vi "create Behaviour.vi"(8 "error in (no error)":errorcluster caption="Fehler (Eingang, kein Fehler)", 11 "TestInterface Eingang":refnum<class "TestInterface.lvclass"> caption="DNL_LabVIEW Object in") -> (0 "error out":errorcluster caption="Fehler (Ausgang)", 1 "regex":string[](array[string]), 2 "response":bool[](array[boolean]), 3 "TestInterface Ausgang":refnum<class "TestInterface.lvclass"> caption="DNL_LabVIEW Object out")   [LabVIEW 2013, in "TestInterface.lvclass"]
doc: "In diesem VI werden die beiden Arrays regex und response für das Verhalten festgelegt. Das Array response definiert, ob eine Antwort auf einen Befehl erwartet wird oder nicht. Die Erstellung des Verhaltens ist hardcoded und wird nicht während der Laufzeit erstellt."
uses:
  TestInterface.lvclass
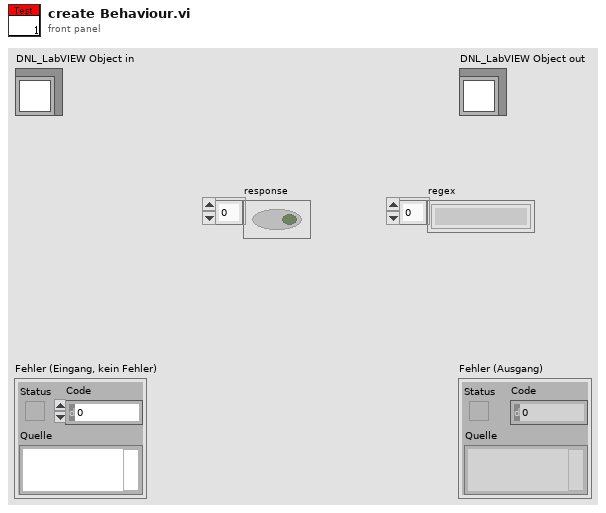
[diagram p1: front panel]
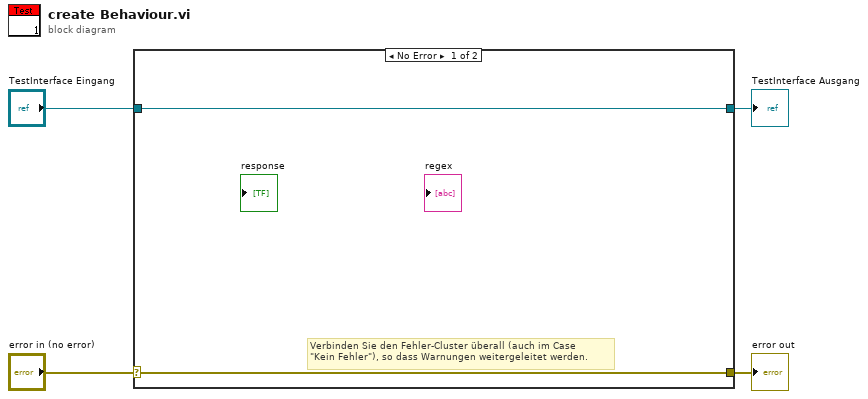
[diagram p0: block diagram]
diagram:
  n1 = case shown="No Error" "error in (no error)" {
    selector: "error in (no error)" -> [w5 w8]
    tunnel: [w5 w8] -> w3
    tunnel: [w6 w7] -> w1
    tunnel: "TestInterface Eingang" -> [w6 w7]
    frame No Error {
      # "Verbinden Sie den Fehler-Cluster überall (auch im Case\n\"Kein Fehler\"), so dass Warnungen weitergeleitet werden."
    }
    frame Error {
    }
  }
  "error out" <- w3
  "TestInterface Ausgang" <- w1
